vi "Expand.vi"(8 "error in (no error)":errorcluster, 10 "ToExpand in":refnum<data-value>, 11 "Tree in":refnum<class "Tree.lvclass">) -> (0 "error out":errorcluster, 1 "ExpandedSearchNodes":refnum<data-value>[](array[refnum]), 2 "ToExpand out":refnum<data-value>, 3 "Tree out":refnum<class "Tree.lvclass">)   [LabVIEW 2013, in "Tree.lvclass"]
doc: "Used to expand our search through the tree. If your tree already has all of its nodes populated then you can use this method as it stands. If the tree is unpopulated or partially populated then you will have create the nodes and out put them through ExpandedSearchNodes. \n\nWarning: Do not link the nodes, the tree class will take care of that. Manually linking nodes may cause search problems."
uses:
  Tree.lvclass
  TreeNode/TreeNode.lvclass
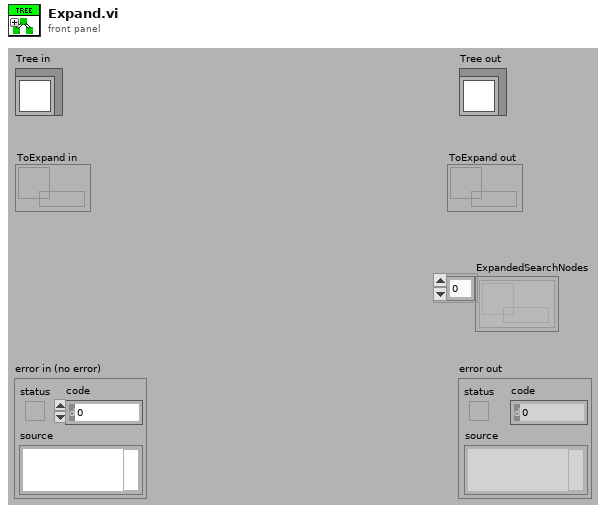
[diagram p1: front panel]
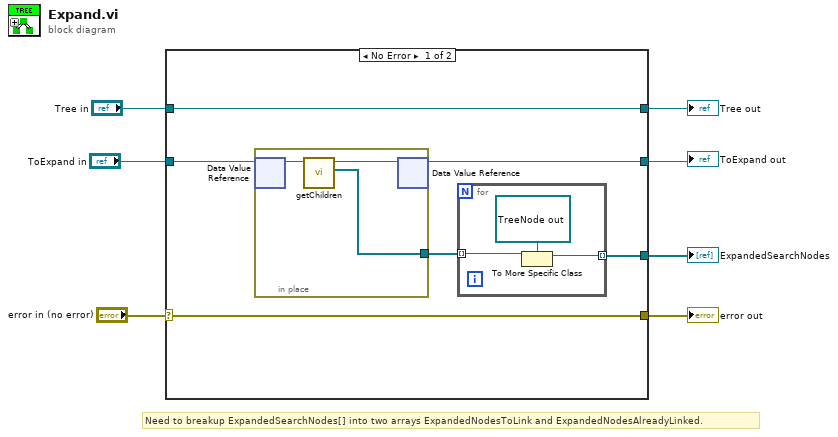
[diagram p0: block diagram]
diagram:
  # "Need to breakup ExpandedSearchNodes[] into two arrays ExpandedNodesToLink and ExpandedNodesAlreadyLinked."
  n1 = case shown="No Error" "error in (no error)" {
    selector: "error in (no error)" -> [w12 w22]
    tunnel: [w12 w22] -> w6
    tunnel: [w13 w21] -> w4
    tunnel: "Tree in" -> [w13 w21]
    tunnel: "ToExpand in" -> [w11 w20]
    tunnel: [w10 w20] -> w2
    tunnel: [w8 _] -> w1
    frame No Error {
      n2 = in-place {
        in-place-border: [w17] -> w9
        n3 = in-place-dvr #1(w11) -> (w19:refnum<class "TreeNode.lvclass">)  [unwired: 1 out]
        n4 = call "getChildren.vi"("TreeNode in"=w19) -> ("Children"=w17:refnum<data-value>[], "TreeNode out"=w18:refnum<class "TreeNode.lvclass">)  [unwired: 8 in, 1 out]
        n5 = in-place-dvr #1(w18) -> (w10:refnum<data-value>)  [unwired: 1 out]
      }
      n6 = for {
        tunnel: w9 -> [w16] mode=indexing
        tunnel: [w14] -> w8 mode=indexing
        n7 = To More Specific Class(target class=refnum<data-value> refnum ("ToExpand in"), reference=w16) -> (specific class reference=w14:refnum<data-value>)  [unwired: 1 in, 1 out]
      }
    }
    frame Error {
    }
  }
  "error out" <- w6
  "Tree out" <- w4
  "ToExpand out" <- w2
  "ExpandedSearchNodes" <- w1
